vi "Main.vi"() -> ()   [LabVIEW 2018]
doc: "This template is for the Queued Message Handler design pattern.\n\nThe Event Handling Loop generates messages based on user interface actions.\n\nThe Message Handling Loop processes messages generated by the Event Handling Loop, or by other messages. The messages are string values, so new messages can be added easily to the Message Cases case structure in the Message Handling Loop. Each message cluster can also provide an optional value for Message Data, which is a variant that can be converted to whatever message-specific data is required."
uses:
  support/mqtt/Controls/QoS.ctl
  support/mqtt/Controls/Retain_Flag.ctl
  support/mqtt/Controls/DUP_Flag.ctl
  support/mqtt/Controls/Connection_Return_Codes.ctl
  controls/UI Data.ctl
  controls/App Data.ctl
  support/viewer/controls/viewewr_bus.ctl
  controls/Subscriber Data.ctl
  controls/Subscriber Comms Refs.ctl
  support/Message Queue/Message Cluster.ctl
  controls/Subscription.ctl
  support/mqtt/Controls/Connect_Flags.ctl
  support/Message Queue/Enqueue Message (Single).vi
  <vilib>/Utility/error.llb/Error Cluster From Error Code.vi
  <vilib>/ErrorRing/Error Ring.xnode
  support/Message Queue/Message Queue.lvlib
  support/User Event - Stop/User Event - Stop.lvlib
  support/mqtt/MQTT_Functions.lvlib
  support/viewer/TopicViewer.lvlib
panel:
  out "String":string
  in  "Combo Box 2":string(combo)="test/CPU/CPUcommand"
  in  "configuration file path":path=path "D:/James Pratice LV/MQTT.ini"
  in  "Key Name":string="Topics"
  in  "Section Name":string="Publish Topic"
  in  "Subscribe  list":string(combo)="test/CPU/CPUcommand"
  in  "Connect Meta":T4={"QoS"=enum."At most once", "DUP"=FALSE, "Retain"=FALSE, "Keep Alive (sec)"=60}
  in  "Tab Control":T5(tab)=enum."Subscribe"
  in  "Command":string="LabVIEW says it's "
  in  "Publish Meta":cluster{"QoS":T1, "Retain":T3, "DUP":T2}
  in  "mqtt_publish":bool
  in  "mqtt|_sendTopic":string="home/garden/fountain"
  out "Message ID (acknowledged)":u16=10
  out "all messge types":string
  in  "Clear Console":bool
  in  "mqtt_unsubscribe":bool
  in  "QoS":T1
  in  "mqtt_subscribeTopic":string(combo)="test/CPU/CPUcommand"
  in  "mqtt_subscribe":bool
  out "Console  - All Topics":string
  out "Active subscriptions":string
  out "unSubID":u16=4
  out "unsubOk":bool=TRUE
  out "subID":u16=2
  out "Granted QoS Levels":T1[](array[typedef])=[enum."At most once", enum."Exactly once", enum."At most once"]
  out "reserved count":i32
  out "Error":bool
  out "Connection Status":T6
  out "Acknowledged":bool
  out "Subscribed":bool
  out "Connected":bool=TRUE
  out "Keep Alive timer sec":dbl=4.544839382171631 caption="Elapsed Time (s)"
  in  "Exit":bool
  out "Last pingresp":bool
  in  "Message Period (ms)":i32=-1 caption="Message Period (ms) - change to -1 to turn off automated messages"
  in  "AM Command":string="LabVIEW says the time is - " caption="Command (will be a prefix to the current system time)"
  in  "AM Topic":string="home/garden/timer" caption="Topic"
  in  "AM Publish Meta":cluster{"QoS":T1, "Retain":T3, "DUP":T2} caption="Publish Meta"
  in  "mqtt_disconnect":bool
  in  "mqtt_connect":bool
  in  "Client ID":string="LVSubscribeClient1"
  in  "port":u16=1883
  in  "address (IP)":string="192.168.86.199"
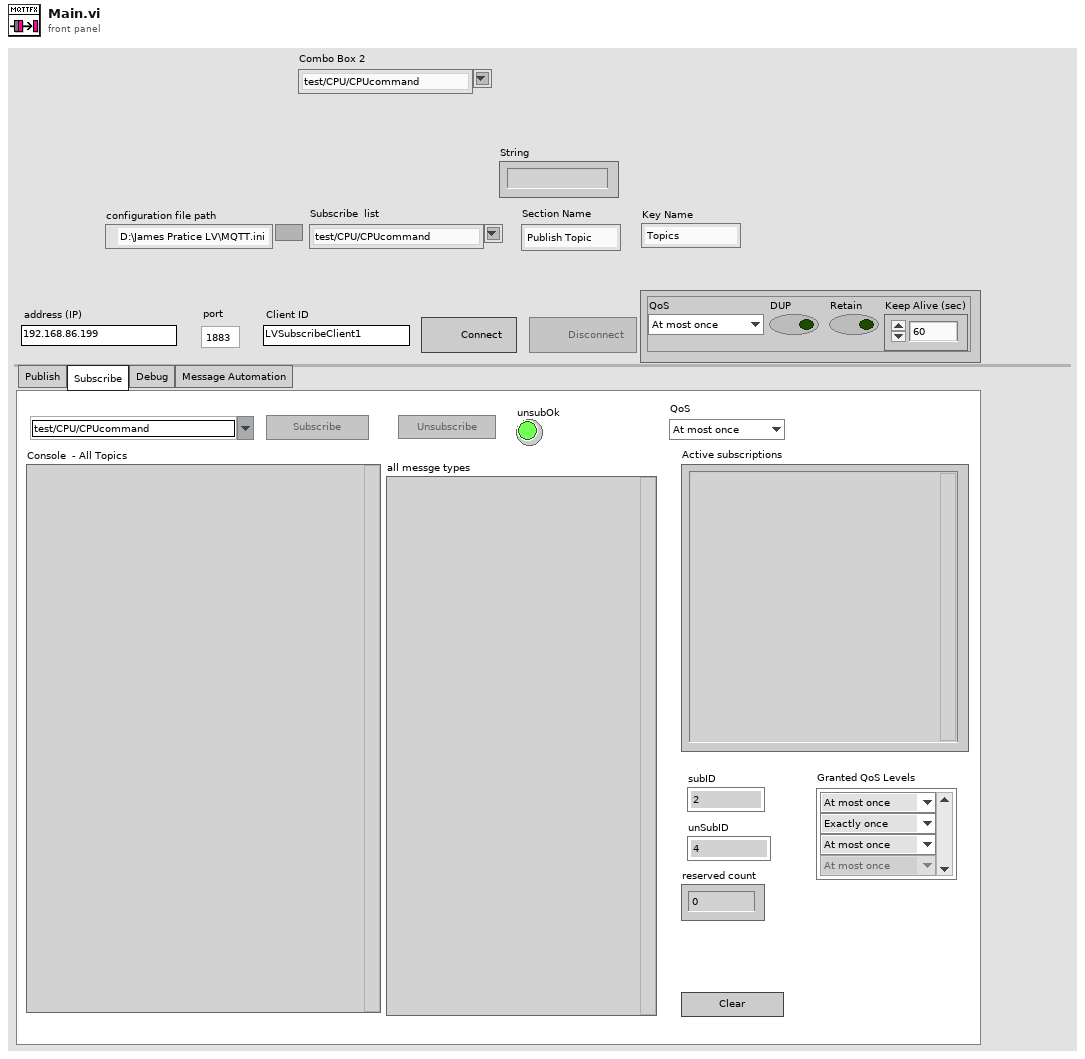
[diagram p1: front panel]
types:
  T1 = typedef "MQTT_Functions.lvlib/QoS.ctl" = enum8{"At most once", "At least once", "Exactly once", "Reserved"}
  T2 = typedef "MQTT_Functions.lvlib/DUP_Flag.ctl" = bool
  T3 = typedef "MQTT_Functions.lvlib/Retain_Flag.ctl" = bool
  T4 = cluster{"QoS":T1, "DUP":T2, "Retain":T3, "Keep Alive (sec)":u16}
  T5 = enum32{"Publish", "Subscribe", "Debug", "Message Automation"}
  T6 = typedef "MQTT_Functions.lvlib/Connection_Return_Codes.ctl" = enum16{"Connection accepted", "Connection refused: unacceptable protocol version", "Connection refused: identifier rejected", "Connection refused: Server unavailable", "Connection refused: bad user name or password", "Connection refused: not authorized"}
  T7 = typedef "Subscriber Comms Refs.ctl" = cluster{"SubscribeQ":refnum<queue>, "Subscriber Notifier":refnum<notifier>}
  T8 = typedef "Subscriber Data.ctl" = cluster{"tcpConnID":refnum<k5>, "subscriptionList":string[], "Subscribed":bool, "Keep Alive (sec)":u16, "Connected":bool, "ViewerRef":T9[], "PacketId":u16}
  T9 = typedef "TopicViewer.lvlib/viewewr_bus.ctl" = cluster{"Topic":refnum<queue>, "Stop":refnum<notifier>, "TopicName":string, "vi reference":refnum<vi>, "StopAck":refnum<notifier>}
  T10 = typedef "App Data.ctl" = cluster{"tcpConnID":refnum<k5>, "subscriptionList":string[], "Connected":bool, "Keep Alive (sec)":u16, "ViewerRef":T9[], "PacketId":u16}
  T11 = typedef "UI Data.ctl" = cluster{"Connect":refnum<vi>, "Disconnect":refnum<vi>, "Subscribe":refnum<vi>, "Unsubscribe":refnum<vi>, "Publish":refnum<vi>}
  T12 = typedef "Message Queue.lvlib/All Message Queues.ctl" = cluster{"UI":refnum<queue>, "SubscribeQ":refnum<queue>}
  T13 = cluster{"connection ID out":refnum<k5>, "Keep Alive (sec)":u16}
  T14 = typedef "TopicViewer.lvlib/Subscription.ctl" = cluster{"subscriptionInfo":cluster{"mqtt_subscribeTopic":string, "QoS":T1}, "ViewerRef":T9}
  T15 = typedef "MQTT_Functions.lvlib/MessageType.ctl" = enum32{"Reserved", "CONNECT", "CONNACK", "PUBLISH", "PUBACK", "PUBREC", "PUBREL", "PUBCOMP", "SUBSCRIBE", "SUBACK", "UNSUBSCRIBE", "UNSUBACK", "PINGREQ", "PINGRESP", "DISCONNECT", "Reserved2"}
  T16 = cluster{"mqtt_subscribeTopic":string, "QoS":T1}[]
  T17 = enum8{"Enabled", "Disabled", "Disabled and Grayed Out"}
  T18 = enum8{"Enabled", "Disabled", "Disabled and Grayed Out"}[]
  T19 = typedef "MQTT_Functions.lvlib/Connect_Flags.ctl" = cluster{"user name":bool, "password":bool, "will retain":bool, "will flag":bool, "clean session":bool, "reserved":bool, "will QoS":T1}
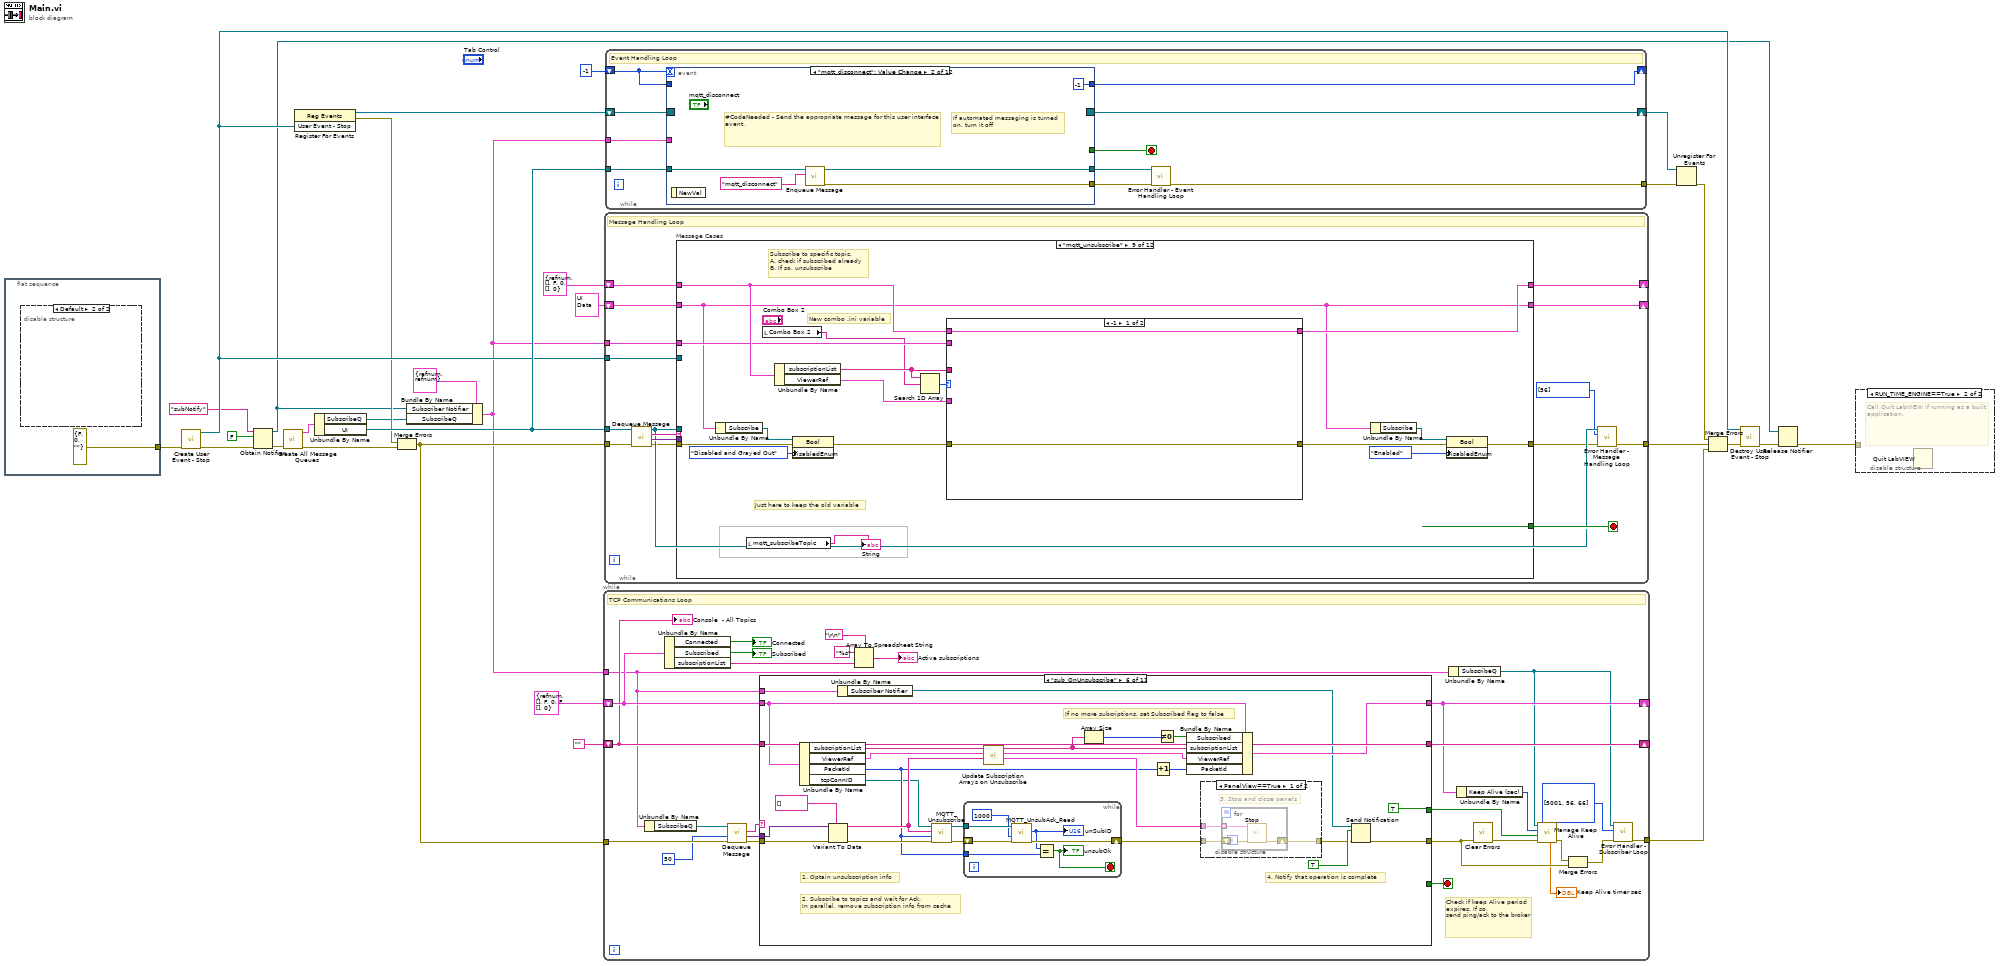
[diagram p0: block diagram]
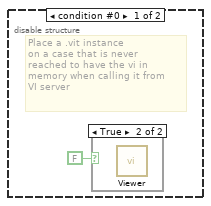
[diagram p2: hidden frame]
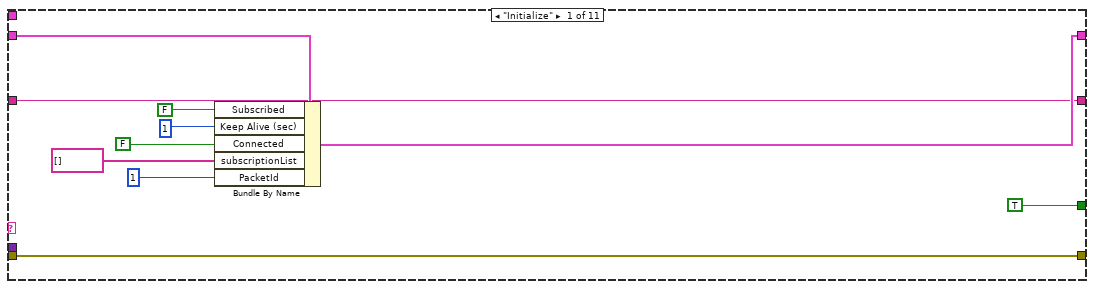
[diagram p4: hidden frame]
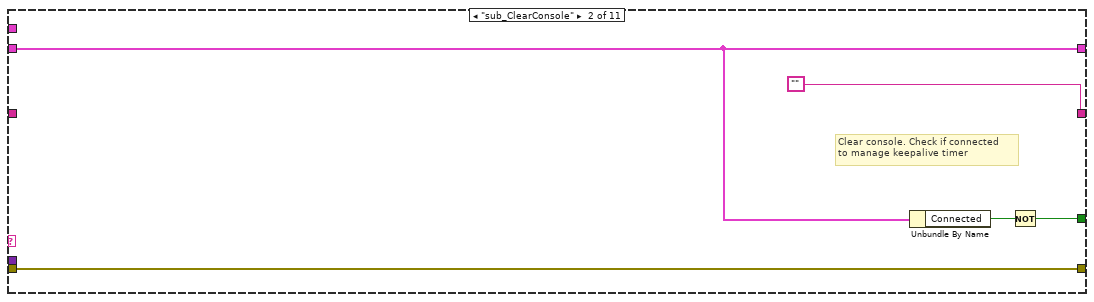
[diagram p5: hidden frame]
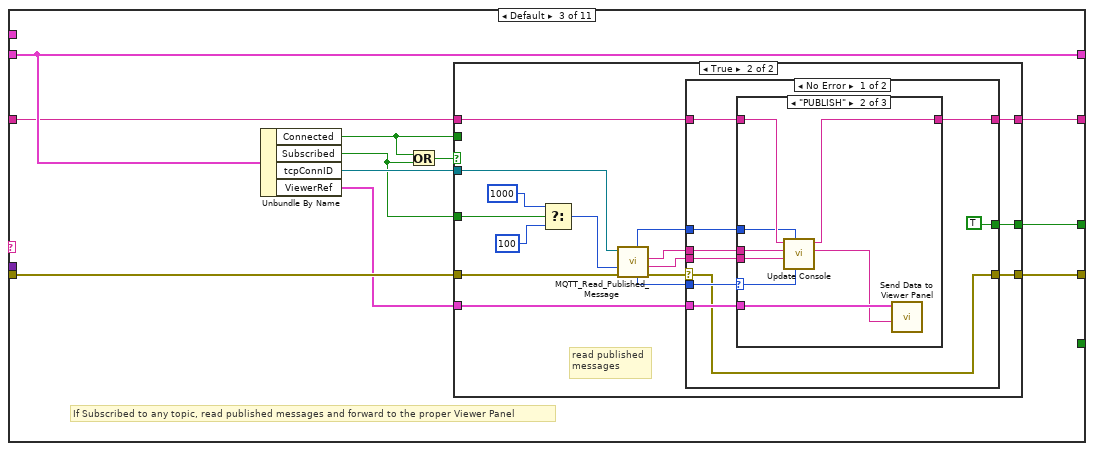
[diagram p6: hidden frame]
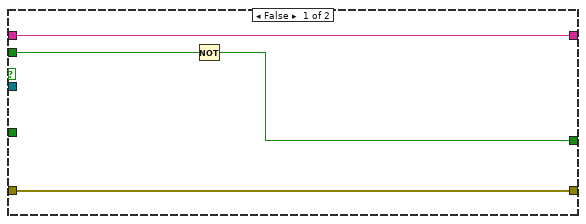
[diagram p7: hidden frame]
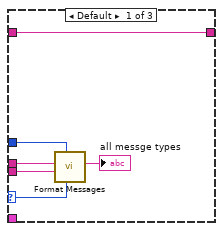
[diagram p8: hidden frame]
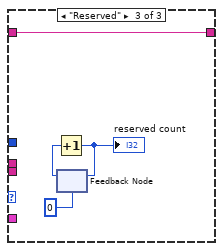
[diagram p9: hidden frame]
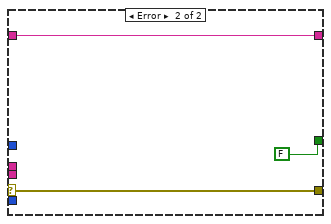
[diagram p10: hidden frame]
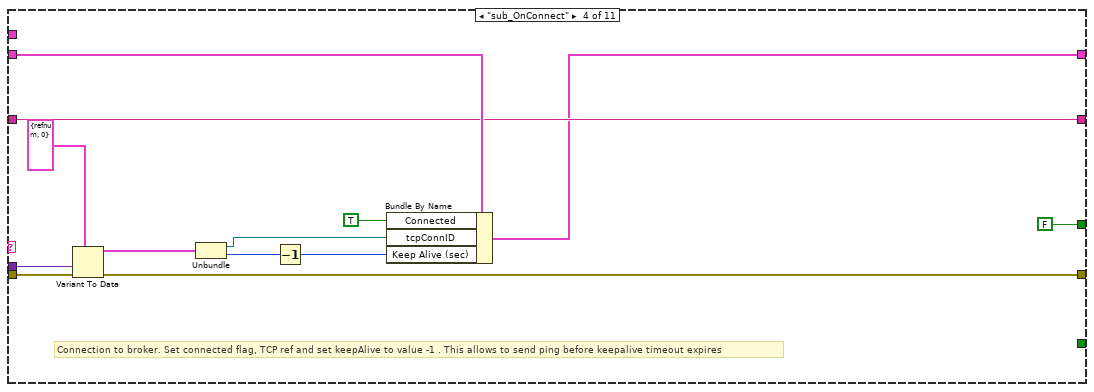
[diagram p11: hidden frame]
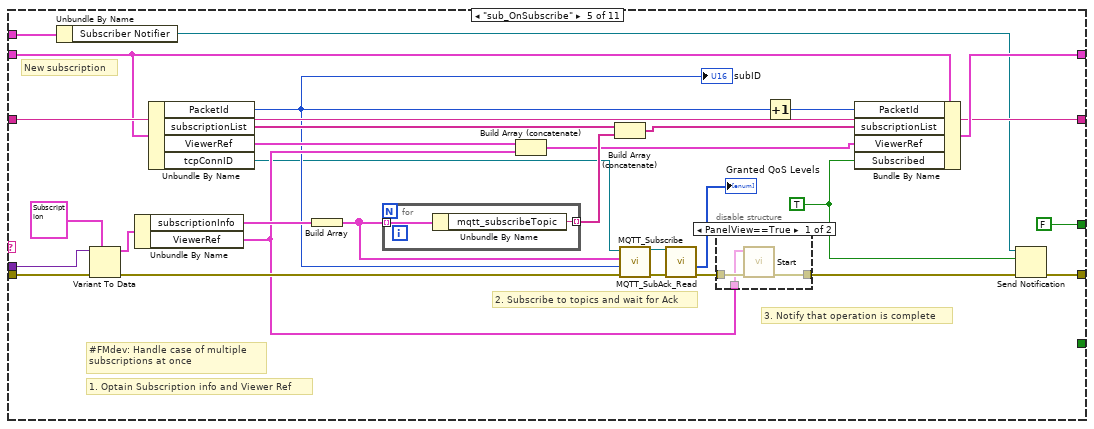
[diagram p12: hidden frame]
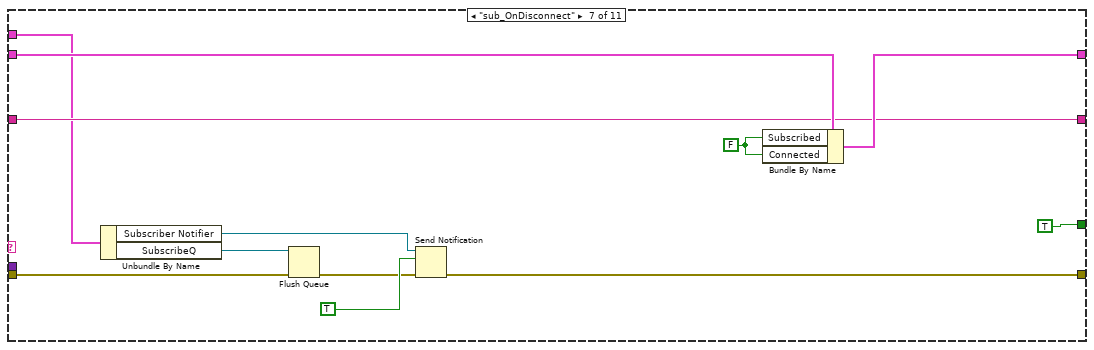
[diagram p15: hidden frame]
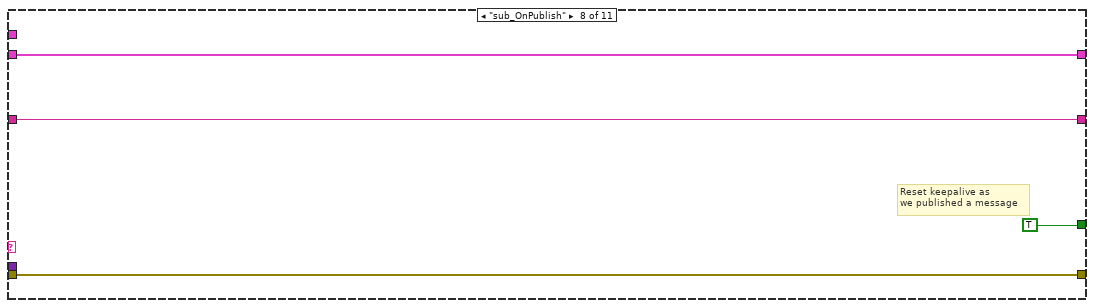
[diagram p16: hidden frame]
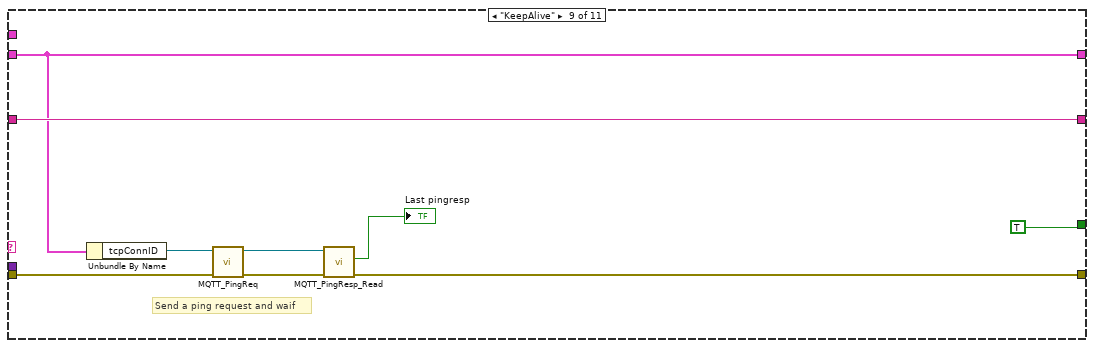
[diagram p17: hidden frame]
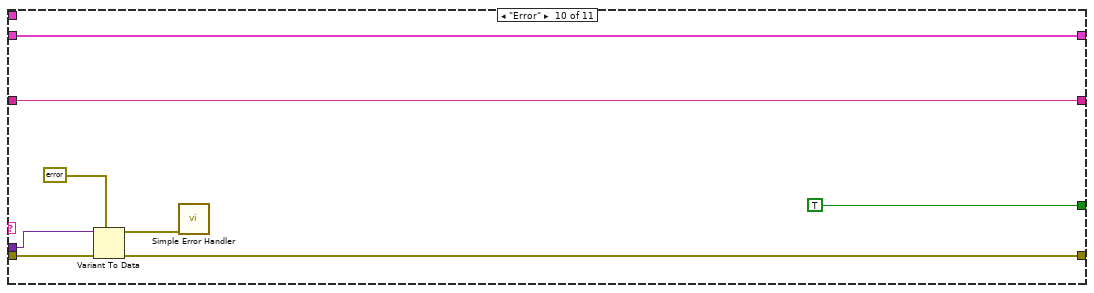
[diagram p18: hidden frame]
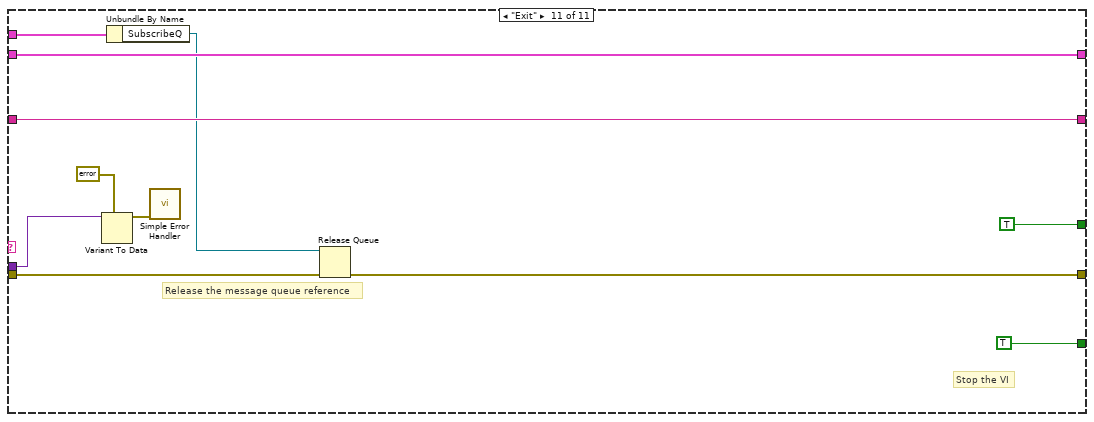
[diagram p19: hidden frame]
diagram:
  n1 = flat-sequence {
    tunnel: [errorcluster {"status"=FALSE, "code"=0, "source"=""} ("error in (no error)")] -> w6
    frame #0 {
      n2 = disable-structure shown="Default" {
        frame condition #0 {
          # "Place a .vit instance \non a case that is never\nreached to have the vi in\nmemory when calling it from \nVI server"
          n3 = case shown="True" FALSE {
            frame False {
            }
            frame True {
              n4 = call "Viewer.vi"() -> ()  [unwired: 11 in, 1 out]
            }
          }
        }
        frame condition #1 (active) {
        }
      }
    }
  }
  n5 = call "Create User Event - Stop.vi"("error in (no error)"=w6) -> ("error out"=w12:errorcluster, "User Event - Stop"=w19:refnum<user-event>)  [unwired: 9 in]
  n6 = Obtain Notifier(name (unnamed)="subNotify", notification data type=FALSE, error in (no error)=w12) -> (notifier out=w5:refnum<notifier>, error out=w11:errorcluster)  [unwired: 1 in, 1 out]
  n7 = call "Create All Message Queues.vi"("error in (no error)"=w11) -> ("error out"=w29:errorcluster, "Message Queues out"=w28:T12)  [unwired: 9 in]
  n8 = register-events(w19) -> (reference out=w20:refnum<event-registration>, error out=w18:errorcluster)  [unwired: 2 in]
  n9 = Unbundle By Name(w28) -> ("SubscribeQ"=w2:refnum<queue>, "UI"=w26:refnum<queue>)
  n10 = Merge Errors(w18, w29) -> (w16:errorcluster)
  n11 = Bundle By Name(cluster=T7 {"SubscribeQ"=refnum, "Subscriber Notifier"=refnum}, "Subscriber Notifier"=w5, "SubscribeQ"=w2) -> (w3:T7)
  n12 = while {
    tunnel: w16 -> [w59]
    shift-right: [w39] -> _
    shift-left: T8 {"tcpConnID"=refnum, "subscriptionList"=[], "Subscribed"=FALSE, "Keep Alive (sec)"=0, "Connected"=FALSE, "ViewerRef"=[], "PacketId"=0} ("App Data") -> [w37]
    tunnel: [w54] -> w14
    shift-right: [w46] -> _
    shift-left: "" -> [w36]
    tunnel: w3 -> [w32]
    stop <- w55 stop-if-true
    # "Check if keep Alive period expires. If so, \nsend ping/ack to the broker"
    # "TCP Communications Loop"
    n13 = Unbundle By Name(w32) -> ("SubscribeQ"=w34:refnum<queue>)
    n14 = Unbundle By Name(w37) -> ("Connected"=→"Connected":bool, "Subscribed"=→"Subscribed":bool, "subscriptionList"=w45:string[])
    n15 = call "Dequeue Message.vi"("error in (no error)"=w59, "timeout in ms (-1)"=50, "Message Queue"=w34) -> ("error out"=w57:errorcluster, "Message Data"=w56:variant, "Message"=w58:string)  [unwired: 5 in, 1 out]
    n16 = case shown="\"sub_OnUnsubscribe\"" w58 {
      tunnel: w57 -> [w68 w74 w83 w146 w171 w209 w233 w237 w248 w254 w264]
      tunnel: w56 -> [_ _ _ w145 w170 w206 _ _ _ w252 w266]
      tunnel: [_ _ _ _ _ _ _ _ _ _ TRUE] -> w55
      tunnel: w37 -> [w69 w72 w85 w148 w168 w200 w236 w240 w247 w257 w263]
      tunnel: [w67 w72 w85 w144 w177 w197 w235 w240 w247 w257 w263] -> w39
      tunnel: [w68 w74 w79 w142 w174 w207 w230 w237 w242 w253 w262] -> w41
      tunnel: w36 -> [w65 _ w82 w147 w176 w210 w234 w239 w249 w251 w261]
      tunnel: [w65 "" w81 w147 w176 w210 w234 w239 w249 w251 w261] -> w46
      tunnel: [TRUE w70 w78 FALSE FALSE TRUE TRUE TRUE TRUE TRUE TRUE] -> w51
      tunnel: w32 -> [_ _ _ _ w150 w185 w227 _ _ _ w259]
      frame "Initialize" {
        n17 = Bundle By Name(cluster=w69, "Subscribed"=FALSE ("Connected"), "Keep Alive (sec)"=u16 1, "Connected"=FALSE, "subscriptionList"=string[] [], "PacketId"=u16 1) -> (w67:T8)
      }
      frame "sub_ClearConsole" {
        # "Clear console. Check if connected\nto manage keepalive timer"
        n18 = Unbundle By Name(w72) -> ("Connected"=w71:bool)
        n19 = Not(x=w71) -> (.not. x?=w70:bool)
      }
      frame Default {
        # "If Subscribed to any topic, read published messages and forward to the proper Viewer Panel"
        n20 = Unbundle By Name(w85) -> ("Connected"=w77:bool, "Subscribed"=w76:bool, "tcpConnID"=w84:refnum<k5>, "ViewerRef"=w80:T9[])
        n21 = Or(x=w77, y=w76) -> (x .or. y?=w75:bool)
        n22 = case shown="True" w75 {
          tunnel: w84 -> [_ w102]
          tunnel: w83 -> [w88 w101]
          tunnel: w82 -> [w89 w100]
          tunnel: [w89 w99] -> w81
          tunnel: [w88 w94] -> w79
          tunnel: w80 -> [_ w98]
          tunnel: [w87 w95] -> w78
          tunnel: w77 -> [w86 _]
          tunnel: w76 -> [_ w93]
          frame False {
            n23 = Not(x=w86) -> (.not. x?=w87:bool)
          }
          frame True {
            # "read published\nmessages"
            n24 = Select(t=1000 ("timeout ms (25000)"), s=w93, f=100 ("timeout ms (25000)")) -> (s? t:f=w90:i32)
            n25 = call "MQTT_Read_Published_Message.vi"("error in (no error)"=w101, "timeout ms (25000)"=w90, "connection ID"=w102) -> ("error out"=w96:errorcluster, "Message"=w104:string, "Topic Name"=w105:string, "MessageType"=w103:T15, "Message ID"=w97:u16)  [unwired: 3 in, 1 out]
            n26 = case shown="No Error" w96 {
              selector: w96 -> [w106 w133]
              tunnel: w105 -> [w114 _]
              tunnel: w104 -> [w113 _]
              tunnel: w103 -> [w112 _]
              tunnel: w100 -> [w111 w134]
              tunnel: [w110 w134] -> w99
              tunnel: w98 -> [w109 _]
              tunnel: w97 -> [w108 _]
              tunnel: [TRUE FALSE] -> w95
              tunnel: [w106 w133] -> w94
              frame No Error {
                n27 = case shown="\"PUBLISH\"" w112 {
                  selector: w112 -> [w116 w121 _]
                  tunnel: w111 -> [w120 w127 w129]
                  tunnel: w114 -> [w119 w124 _]
                  tunnel: w113 -> [w118 w123 _]
                  tunnel: [w120 w126 w129] -> w110
                  tunnel: w109 -> [_ w128 _]
                  tunnel: w108 -> [w115 w122 _]
                  frame Default {
                    n28 = call "Format Messages.vi"("MessageType"=w116, "Message ID"=w115, "Message"=w118, "Topic Name"=w119) -> ("Message String"=→"all messge types":string)  [unwired: 7 in]
                  }
                  frame "PUBLISH" {
                    n29 = call "Update Console.vi"("MessageType"=w121, "Message ID"=w122, "Message"=w123, "Topic Name"=w124, "Console In"=w127) -> ("Message String"=w125:string, "Console Out"=w126:string)  [unwired: 5 in]
                    n30 = call "Send Data to Viewer Panel.vi"("Message String"=w125, "ViewerRef Array"=w128) -> ()  [unwired: 10 in]
                  }
                  frame "Reserved" {
                    n31 = feedback #1(0) -> (w131:i32)
                    n32 = Increment(x=w131) -> (x+1=w130:i32)
                    "reserved count" <- w130
                    n33 = feedback-in #1(w130) -> ()
                  }
                }
              }
              frame Error {
              }
            }
          }
        }
      }
      frame "sub_OnConnect" {
        # "Connection to broker. Set connected flag, TCP ref and set keepAlive to value -1 . This allows to send ping before keepalive timeout expires"
        n34 = Variant To Data(error in=w146, type=T13 {"connection ID out"=refnum, "Keep Alive (sec)"=0} ("output cluster"), Variant=w145) -> (data=w139:T13, error out=w142:errorcluster)
        n35 = Unbundle(w139) -> ("connection ID out"=w138:refnum<k5>, "Keep Alive (sec)"=w137:u16)
        n36 = Decrement(x=w137) -> (x-1=w136:u16)
        n37 = Bundle By Name(cluster=w148, "Connected"=TRUE, "tcpConnID"=w138, "Keep Alive (sec)"=w136) -> (w144:T8)
      }
      frame "sub_OnSubscribe" {
        w154 = TRUE ("notification")
        # "3. Notify that operation is complete"
        # "2. Subscribe to topics and wait for Ack"
        # "#FMdev: Handle case of multiple\nsubscriptions at once"
        # "1. Optain Subscription info and Viewer Ref"
        # "New subscription"
        n38 = Unbundle By Name(w150) -> ("Subscriber Notifier"=w149:refnum<notifier>)
        n39 = Variant To Data(error in=w171, type=T14 {"subscriptionInfo"={"mqtt_subscribeTopic"="", "QoS"=enum."At most once"}, "ViewerRef"={"Topic"=refnum, "Stop"=refnum, "TopicName"="", "vi reference"=refnum, "StopAck"=refnum}}, Variant=w170) -> (data=w163:T14, error out=w169:errorcluster)
        n40 = Unbundle By Name(w163) -> ("subscriptionInfo"=w162:cluster{"mqtt_subscribeTopic":string, "QoS":T1}, "ViewerRef"=w157:T9)
        n41 = Unbundle By Name(w168) -> ("PacketId"=w153:u16, "subscriptionList"=w167:string[], "ViewerRef"=w160:T9[], "tcpConnID"=w151:refnum<k5>)
        "subID" <- w153
        n42 = Build Array(w162) -> (w161:T16)
        n43 = for {
          tunnel: w161 -> [w183] mode=indexing
          tunnel: [w182] -> w166 mode=indexing
          n44 = Unbundle By Name(w183) -> ("mqtt_subscribeTopic"=w182:string)
        }
        n45 = Build Array (concatenate)(w160, w157) -> (w159:T9[])
        n46 = Build Array (concatenate)(w167, w166) -> (w165:string[])
        n47 = call "MQTT_Subscribe.vi"("error in (no error)"=w169, "Message ID"=w153, "Subscription Info Array"=w161, "connection ID"=w151) -> ("error out"=w173:errorcluster, "connection ID out"=w172:refnum<k5>)  [unwired: 6 in]
        n48 = call "MQTT_SubAck_Read.vi"("error in (no error)"=w173, "connection ID"=w172) -> ("error out"=w158:errorcluster, "Granted QoS Levels"=→"Granted QoS Levels":T1[])  [unwired: 7 in, 1 out]
        n49 = disable-structure shown="PanelView==True" {
          disable-tunnel: w158 -> [w180 w181]
          disable-tunnel: w157 -> [w179 _]
          disable-tunnel: [w178 w181] -> w156
          frame condition #0 {
            n50 = call "Start.vi"("error in (no error)"=w180, "ViewerRef"=w179) -> ("error out"=w178:errorcluster)  [unwired: 9 in]
          }
          frame condition #1 (active) {
          }
        }
        n51 = Increment(x=w153) -> (x+1=w152:u16)
        n52 = Bundle By Name(cluster=w168, "PacketId"=w152, "subscriptionList"=w165, "ViewerRef"=w159, "Subscribed"=w154) -> (w177:T8)
        n53 = Send Notification(notification=w154, notifier=w149, error in (no error)=w156) -> (error out=w174:errorcluster)  [unwired: 1 out]
      }
      frame "sub_OnUnsubscribe" {
        # "If no more subcriptions, set Subscribed flag to false"
        # "2. Subscribe to topics and wait for Ack.\nIn parallel, remove subscription info from cache"
        # "1. Optain unsubscription info"
        # "4. Notify that operation is complete"
        n54 = Unbundle By Name(w200) -> ("subscriptionList"=w202:string[], "ViewerRef"=w188:T9[], "PacketId"=w189:u16, "tcpConnID"=w186:refnum<k5>)
        n55 = Variant To Data(error in=w209, type=string[] [] ("UnSubscribe Topic Array"), Variant=w206) -> (data=w201:string[], error out=w190:errorcluster)
        n56 = Unbundle By Name(w185) -> ("Subscriber Notifier"=w184:refnum<notifier>)
        n57 = call "MQTT_Unsubscribe.vi"("error in (no error)"=w190, "Message ID"=w189, "UnSubscribe Topic Array"=w201, "connection ID"=w186) -> ("error out"=w205:errorcluster, "connection ID out"=w204:refnum<k5>)  [unwired: 5 in, 1 out]
        n58 = while {
          tunnel: w204 -> [w216]
          tunnel: w189 -> [w212]
          shift-right: [w214] -> w194
          shift-left: w205 -> [w217]
          stop <- w211 stop-if-true
          n59 = call "MQTT_UnsubAck_Read.vi"("error in (no error)"=w217, "timeout ms (25000)"=1000, "connection ID"=w216) -> ("error out"=w214:errorcluster, "MessageID"=w213:u16)  [unwired: 6 in, 1 out]
          "unSubID" <- w213
          n60 = Equal?(x=w213, y=w212) -> (x = y?=w211:bool)
          "unsubOk" <- w211
        }
        n61 = call "Update Subscription Arrays on Unsubscribe.vi"("UnSubscribe Topic Array"=w201, "ViewerRef in"=w188, "subscriptionList in"=w202) -> ("ViewerRef's to close"=w192:T9[], "ViewerRef out"=w195:T9[], "subscriptionList out"=w199:string[])  [unwired: 6 in]
        n62 = Array Size(array=w199) -> (size(s)=w198:i32)
        n63 = Increment(x=w189) -> (x+1=w191:u16)
        n64 = Not Equal To 0?(x=w198) -> (x != 0?=w187:bool)
        n65 = Bundle By Name(cluster=w200, "Subscribed"=w187, "subscriptionList"=w199, "ViewerRef"=w195, "PacketId"=w191) -> (w197:T8)
        n66 = disable-structure shown="PanelView==True" {
          disable-tunnel: w194 -> [w220 w224]
          disable-tunnel: [w219 w224] -> w193
          disable-tunnel: w192 -> [w218 _]
          frame condition #0 {
            # "3. Stop and close panels"
            n67 = for {
              tunnel: w218 -> [w221] mode=indexing
              shift-right: [w222] -> w219
              shift-left: w220 -> [w223]
              n68 = call "Stop.vi"("error in (no error)"=w223, "ViewerRef"=w221) -> ("error out"=w222:errorcluster)  [unwired: 9 in]
            }
          }
          frame condition #1 (active) {
          }
        }
        n69 = Send Notification(notification=TRUE, notifier=w184, error in (no error)=w193) -> (error out=w207:errorcluster)  [unwired: 1 out]
      }
      frame "sub_OnDisconnect" {
        w228 = FALSE ("Subscribed")
        n70 = Unbundle By Name(w227) -> ("Subscriber Notifier"=w226:refnum<notifier>, "SubscribeQ"=w225:refnum<queue>)
        n71 = Flush Queue(queue=w225, error in (no error)=w233) -> (error out=w231:errorcluster)  [unwired: 2 out]
        n72 = Send Notification(notification=TRUE, notifier=w226, error in (no error)=w231) -> (error out=w230:errorcluster)  [unwired: 1 out]
        n73 = Bundle By Name(cluster=w236, "Subscribed"=w228, "Connected"=w228) -> (w235:T8)
      }
      frame "sub_OnPublish" {
        # "Reset keepalive as \nwe published a message"
      }
      frame "KeepAlive" {
        # "Send a ping request and waif"
        n74 = Unbundle By Name(w247) -> ("tcpConnID"=w246:refnum<k5>)
        n75 = call "MQTT_PingReq.vi"("error in (no error)"=w248, "connection ID"=w246) -> ("error out"=w243:errorcluster, "connection ID out"=w244:refnum<k5>)  [unwired: 7 in, 1 out]
        n76 = call "MQTT_PingResp_Read.vi"("error in (no error)"=w243, "connection ID"=w244) -> ("error out"=w242:errorcluster, "ok"=→"Last pingresp":bool)  [unwired: 7 in, 1 out]
      }
      frame "Error" {
        n77 = Variant To Data(error in=w254, type=errorcluster {"status"=FALSE, "code"=0, "source"=""} ("error constant"), Variant=w252) -> (data=w256:errorcluster, error out=w253:errorcluster)
        n78 = call <vilib>:"Simple Error Handler.vi"("error in (no error)"=w256) -> ()  [unwired: 4 in, 5 out]
      }
      frame "Exit" {
        # "Release the message queue reference"
        # "Stop the VI"
        n79 = Variant To Data(type=errorcluster {"status"=FALSE, "code"=0, "source"=""} ("error constant"), Variant=w266) -> (data=w267:errorcluster)  [unwired: 1 in, 1 out]
        n80 = Unbundle By Name(w259) -> ("SubscribeQ"=w258:refnum<queue>)
        n81 = call <vilib>:"Simple Error Handler.vi"("error in (no error)"=w267) -> ()  [unwired: 4 in, 5 out]
        n82 = Release Queue(queue=w258, error in (no error)=w264) -> (error out=w262:errorcluster)  [unwired: 1 in, 2 out]
      }
    }
    n83 = Array To Spreadsheet String(delimiter (Tab)="\r\n", array=w45, 3:"%s" ("format string")) -> (spreadsheet string=→"Active subscriptions":string)
    n84 = Unbundle By Name(w32) -> ("SubscribeQ"=w33:refnum<queue>)
    n85 = Unbundle By Name(w39) -> ("Keep Alive (sec)"=w38:u16)
    n86 = call <vilib>:"Clear Errors.vi"("error in (no error)"=w41) -> ("error out"=w44:errorcluster)  [unwired: 5 in, 1 out]
    n87 = call "Manage Keep Alive.vi"("error in (no error)"=w44, "Reset Keepalive"=w51, "Keep Alive (sec)"=w38, "SubscriberQ"=w33) -> ("error out"=w43:errorcluster, "Elapsed Time (s)"=→"Keep Alive timer sec":dbl)  [unwired: 6 in]
    n88 = Merge Errors(w43, w41) -> (w42:errorcluster)
    n89 = call "Error Handler - Subscriber Loop.vi"("error in (no error)"=w42, "Ignore Errors (Runtime)"=i32[] [5001, 56, 66], "Message Queue"=w33) -> ("dup error in"=w54:errorcluster)  [unwired: 7 in, 1 out]
    "Console  - All Topics" <- w36
  }
  n90 = while {
    tunnel: w26 -> [w277]
    shift-right: [w283] -> _
    shift-left: T11 {"Connect"=refnum, "Disconnect"=refnum, "Subscribe"=refnum, "Unsubscribe"=refnum, "Publish"=refnum} ("Data Cluster") -> [w284]
    tunnel: w19 -> [w281]
    tunnel: w16 -> [w280]
    tunnel: [w275] -> w27
    shift-right: [w272] -> _
    shift-left: T10 {"tcpConnID"=refnum, "subscriptionList"=[], "Connected"=FALSE, "Keep Alive (sec)"=0, "ViewerRef"=[], "PacketId"=0} -> [w273]
    tunnel: w3 -> [w269]
    stop <- w282 stop-if-true
    # "Message Handling Loop"
    n91 = call "Dequeue Message.vi"("error in (no error)"=w280, "Message Queue"=w277) -> ("error out"=w270:errorcluster, "Message Data"=w278:variant, "Message"=w279:string, "dup Message Queue"=w276:refnum<queue>)  [unwired: 6 in]
    n92 = case "Message Cases" shown="\"mqtt_unsubscribe\"" w279 {
      selector: w279 -> [_ _ _ _ _ _ _ _ _ _ _ w571]
      tunnel: w276 -> [_ _ _ w324 _ _ _ _ _ _ w569 _]
      tunnel: w270 -> [w288 w306 w316 w323 w349 w397 w423 w454 w502 w540 w562 _]
      tunnel: [w287 w304 w310 w322 w334 w386 w414 w457 w494 w536 w565 w572] -> w274
      tunnel: w284 -> [w301 w308 w315 w325 w340 w389 w425 w453 w493 w541 w568 w573]
      tunnel: [w289 w308 w315 w325 w339 w389 w425 w452 w493 w541 w568 w573] -> w283
      tunnel: [_ _ _ _ _ _ _ _ _ _ TRUE _] -> w282
      tunnel: w278 -> [_ _ w314 _ _ _ _ _ _ _ w559 _]
      tunnel: w281 -> [_ _ _ _ _ _ _ _ _ _ w564 _]
      tunnel: w273 -> [w300 w307 w309 w321 w341 w384 w424 w459 w507 w539 w558 w570]
      tunnel: [w299 w307 w309 w321 w342 w396 w411 w458 w506 w538 w558 w570] -> w272
      tunnel: w269 -> [_ w303 _ _ w333 w385 w406 w451 w501 w533 _ _]
      frame "Initialize" {
        w285 = T18 [enum."Enabled", enum."Disabled and Grayed Out", enum."Disabled and Grayed Out", enum."Disabled and Grayed Out", enum."Disabled and Grayed Out"] items=["Enabled", "Disabled", "Disabled and Grayed Out"] ("State Array")
        w286 = ""
        w291 = FALSE ("Subscribed")
        # "Initialize local variables"
        # "Initialize buttons"
        # "#FMdev: 1) Vi server to manage UI"
        # "Initialize - All initialization work should take place in this message, since other loops can potentially enqueue messages that execute immediately after this one."
        n93 = control-ref of="mqtt_connect"() -> (w297:refnum<vi>)
        n94 = control-ref of="mqtt_disconnect"() -> (w296:refnum<vi>)
        n95 = control-ref of="mqtt_subscribe"() -> (w295:refnum<vi>)
        n96 = control-ref of="mqtt_unsubscribe"() -> (w294:refnum<vi>)
        n97 = control-ref of="mqtt_publish"() -> (w292:refnum<vi>)
        n98 = Bundle By Name(cluster=w301, "Connect"=w297, "Disconnect"=w296, "Subscribe"=w295, "Unsubscribe"=w294, "Publish"=w292) -> (w289:T11)
        n99 = Bundle By Name(cluster=w300, "Connected"=FALSE, "subscriptionList"=string[] [], "PacketId"=u16 1) -> (w299:T10)
        n100 = local write "Console  - All Topics"(w286) -> ()
        n101 = local write "Active subscriptions"(w286) -> ()
        n102 = local write "Last pingresp"(w291) -> ()
        n103 = local write "Connected"(w291) -> ()
        n104 = local write "Subscribed"(w291) -> ()
        n105 = local write "Error"(w291) -> ()
        n106 = call "Enable Disable Controls.vi"("error in (no error)"=w288, "State Array"=w285, "Data Cluster"=w289) -> ("error out"=w287:errorcluster)  [unwired: 8 in]
      }
      frame "ClearConsole" {
        # "Proxy to clear console from old messages"
        n107 = Unbundle By Name(w303) -> ("SubscribeQ"=w302:refnum<queue>)
        n108 = call-poly "Enqueue Message.vi"("error in (no error)"=w306, "Message"="sub_ClearConsole", "Message Queue"=w302) -> ("error out"=w304:errorcluster)  [unwired: 7 in, 1 out]
      }
      frame "Error" {
        # "#CodeRecommended - If you ever change the name of this \"Error\" message, you'll need to update the name in the Check Loop Error.vi as well."
        # "#CodeRecommended - Consider creating a system for logging errors in some way. These errors are for notification purposes only. Handling of specific errors should be performed in the message frames that generated the error."
        # "Error - Display an error dialog. This message is sent by the \"Error Handler\" VIs at the end of other loops in this application."
        n109 = Variant To Data(error in=w316, type=errorcluster {"status"=FALSE, "code"=0, "source"=""} ("error constant"), Variant=w314) -> (data=w312:errorcluster, error out=w311:errorcluster)
        n110 = call <vilib>:"Simple Error Handler.vi"("error in (no error)"=w312) -> ()  [unwired: 4 in, 5 out]
        n111 = Merge Errors(w311) -> (w310:errorcluster)
      }
      frame "Confirm Quit" {
        # "If connected to a broker, then unsubcribe to existing topics and disconnect\nIf not connected, just exit"
        # "Confirm Quit - Message that can confirm whether or not the user wants to exit the application."
        n112 = Unbundle By Name(w321) -> ("Connected"=w320:bool)
        n113 = Select(t=string[] ["mqtt_unsubscribeAll", "mqtt_disconnect", "Exit"] ("Message"), s=w320, f=string[] ["Exit"]) -> (s? t:f=w319:string[])
        n114 = for {
          tunnel: w319 -> [w326] mode=indexing
          shift-right: [w328] -> w322
          shift-left: w323 -> [w329]
          tunnel: w324 -> [w327]
          n115 = call-poly "Enqueue Message.vi"("error in (no error)"=w329, "Message"=w326, "Message Queue"=w327) -> ("error out"=w328:errorcluster)  [unwired: 7 in, 1 out]
        }
      }
      frame "mqtt_connect" {
        w348 = T19 {"user name"=FALSE, "password"=FALSE, "will retain"=FALSE, "will flag"=FALSE, "clean session"=FALSE, "reserved"=FALSE, "will QoS"=enum."At most once"}  # Connect Flags
        # "Filter on error and then on connection status"
        # "Connect to broker using user provided\nvalue. Using default collect flags"
        n116 = Bundle("address (IP)"="address (IP)", "port"="port") -> (w344:cluster{"address (IP)":string, "port":u16})  [unwired: 1 in]
        n117 = call "MQTT_Connect.vi"("timeout ms (20000)"=10000, "Connect Meta"="Connect Meta", "Client ID"="Client ID", "Connect Flags"=w348, "error in (no error)"=w349, "MQTT Broker"=w344) -> ("error out"=w336:errorcluster, "Connection Status"=w343:T6, "connection ID out"=w331:refnum<k5>)  [unwired: 3 in]
        "Connection Status" <- w343
        n118 = Unbundle By Name("Connect Meta") -> ("Keep Alive (sec)"=w330:u16)
        n119 = Unbundle By Name(w333) -> ("SubscribeQ"=w332:refnum<queue>)
        n120 = case shown="No Error" w336 {
          selector: w336 -> [w354 w382]
          tunnel: w343 -> [w360 _]
          tunnel: [w359 w381] -> w342
          tunnel: w341 -> [w358 w381]
          tunnel: w340 -> [w357 w380]
          tunnel: [w356 w380] -> w339
          tunnel: w330 -> [w355 _]
          tunnel: [w351 w382] -> w334
          tunnel: [w353 TRUE ("Timeout")] -> w335
          tunnel: w332 -> [w352 _]
          tunnel: w331 -> [w350 _]
          frame No Error {
            n121 = case shown="\"Connection accepted\", Default" w360 {
              tunnel: w358 -> [w374 w378]
              tunnel: [w373 w378] -> w359
              tunnel: w357 -> [w371 w377]
              tunnel: [w371 w377] -> w356
              tunnel: w355 -> [w362 _]
              tunnel: w354 -> [w368 w376]
              tunnel: [w364 w376] -> w351
              tunnel: [FALSE ("Timeout") TRUE ("Timeout")] -> w353
              tunnel: w352 -> [w367 _]
              tunnel: w350 -> [w363 _]
              frame "Connection accepted", Default {
                w366 = T18 [enum."Disabled and Grayed Out", enum."Enabled", enum."Enabled", enum."Disabled and Grayed Out", enum."Enabled"] items=["Enabled", "Disabled", "Disabled and Grayed Out"] ("State Array")
                # "Connection accepted, change UI accordingly and send OnConnect event to\nSubscriber Loop"
                n122 = Bundle By Name(cluster=w374, "Connected"=TRUE, "Keep Alive (sec)"=w362, "tcpConnID"=w363) -> (w373:T10)
                n123 = Bundle("connection ID out"=w363, "Keep Alive (sec)"=w362) -> (w361:T13)  [unwired: 1 in]
                n124 = call-poly "Enqueue Message.vi"("error in (no error)"=w368, "Message Data"=w361, "Message"="sub_OnConnect", "Message Queue"=w367) -> ("error out"=w365:errorcluster)  [unwired: 6 in, 1 out]
                n125 = call "Enable Disable Controls.vi"("error in (no error)"=w365, "State Array"=w366, "Data Cluster"=w371) -> ("error out"=w364:errorcluster)  [unwired: 8 in]
              }
              frame "Connection refused: unacceptable protocol version" {
                # "#FM_note: manage refused connection"
              }
            }
          }
          frame Error {
            # "Error connecting. Filter specific errors later on Error Handler VI later on"
          }
        }
        "Error" <- w335
      }
      frame "mqtt_disconnect" {
        w388 = T18 [enum."Enabled", enum."Disabled and Grayed Out", enum."Disabled and Grayed Out", enum."Disabled and Grayed Out", enum."Disabled and Grayed Out"] items=["Enabled", "Disabled", "Disabled and Grayed Out"] ("State Array")
        # "Disconnect anyway and change UI accordingly"
        # "Send OnDisconnect message to subscriber loop and \nwait for operation completed (notifier received)"
        n126 = Unbundle By Name(w384) -> ("subscriptionList"=w383:string[])
        n127 = Unbundle By Name(w384) -> ("tcpConnID"=w398:refnum<k5>)
        n128 = Array Size(array=w383) -> (size(s)=w395:i32)
        n129 = case shown="0" w395 {
          tunnel: w397 -> [w399 w404]
          tunnel: [w399 w403] -> w394
          tunnel: w383 -> [_ w400]
          tunnel: w385 -> [_ w402]
          frame 0 {
          }
          frame Default {
            n130 = call "Send Msg and Wait on Response.vi"("error in (no error)"=w404, "Message Data"=w400, "Message"="sub_OnUnsubscribe", "Subscription References"=w402) -> ("error out"=w403:errorcluster)  [unwired: 7 in]
          }
        }
        n131 = call "Send Msg and Wait on Response.vi"("error in (no error)"=w394, "Message"="sub_OnDisconnect", "Subscription References"=w385) -> ("error out"=w393:errorcluster)  [unwired: 8 in]
        n132 = Bundle By Name(cluster=w384, "Connected"=FALSE, "subscriptionList"=string[] []) -> (w396:T10)
        n133 = call "MQTT_Disconnect.vi"("error in (no error)"=w393, "connection ID"=w398) -> ("error out"=w387:errorcluster)  [unwired: 9 in]
        n134 = call "Enable Disable Controls.vi"("error in (no error)"=w387, "State Array"=w388, "Data Cluster"=w389) -> ("error out"=w386:errorcluster)  [unwired: 8 in]
      }
      frame "mqtt_publish" {
        # "Send an OnPublish message to\nreset keepAlive counter on subcriber"
        # "Publish message. Depending on Quality of Service, handle ack signals"
        n135 = Unbundle By Name(w424) -> ("tcpConnID"=w422:refnum<k5>, "PacketId"=w412:u16)
        n136 = call "MQTT_Publish.vi"("Message ID"=w412, "Publish Meta"="Publish Meta", "error in (no error)"=w423, "Message to be published"="Command", "Topic"="mqtt|_sendTopic", "connection ID"=w422) -> ("error out"=w419:errorcluster, "connection ID out"=w418:refnum<k5>)  [unwired: 4 in]
        n137 = Unbundle By Name("Publish Meta") -> ("QoS"=w420:T1)
        n138 = Unbundle By Name(w406) -> ("SubscribeQ"=w405:refnum<queue>)
        n139 = case shown="\"At most once\", Default" w420 {
          tunnel: w419 -> [w428 w433 w444]
          tunnel: w418 -> [_ w434 w445]
          tunnel: [w428 w431 w438] -> w415
          tunnel: w412 -> [w426 w432 w443]
          tunnel: [FALSE w430 w439] -> w410
          tunnel: [w426 w429 w437] -> w408
          frame "At most once", Default {
            # "QoS 0: no PubACK, fire and forget"
          }
          frame "At least once" {
            # "QoS 1: PubACK"
            n140 = call "MQTT_PubAck_Read.vi"("error in (no error)"=w433, "connection ID"=w434) -> ("error out"=w431:errorcluster, "Message ID"=w429:u16)  [unwired: 7 in, 1 out]
            n141 = Equal?(x=w429, y=w432) -> (x = y?=w430:bool)
          }
          frame "Exactly once" {
            # "QoS 2: PubREC, PubREL, PubCOMP"
            n142 = call "MQTT_PubRec_Read.vi"("error in (no error)"=w444, "connection ID"=w445) -> ("error out"=w442:errorcluster, "Message ID"=w440:u16, "connection ID out"=w441:refnum<k5>)  [unwired: 7 in]
            n143 = call "MQTT_PubRel_Send.vi"("error in (no error)"=w442, "Message ID"=w440, "connection ID"=w441) -> ("error out"=w435:errorcluster, "connection ID out"=w436:refnum<k5>)  [unwired: 6 in, 1 out]
            n144 = call "MQTT_PubComp_Read.vi"("error in (no error)"=w435, "connection ID"=w436) -> ("error out"=w438:errorcluster, "Message ID"=w437:u16)  [unwired: 7 in, 1 out]
            n145 = Equal?(x=w437, y=w443) -> (x = y?=w439:bool)
          }
        }
        "Message ID (acknowledged)" <- w408
        "Acknowledged" <- w410
        n146 = Increment(x=w408) -> (x+1=w407:u16)
        n147 = Select(t=w407, s=w410, f=w408) -> (s? t:f=w409:u16)
        n148 = Bundle By Name(cluster=w424, "PacketId"=w409) -> (w411:T10)
        n149 = call-poly "Enqueue Message.vi"("error in (no error)"=w415, "Message"="sub_OnPublish", "Message Queue"=w405) -> ("error out"=w414:errorcluster)  [unwired: 7 in, 1 out]
      }
      frame "mqtt_subscribe" {
        n150 = control-ref of="Subscribe  list"() -> (w447:refnum<vi>)
        n151 = call "Fill_Combo_API_Box (SubVI).vi"("Section Name"="Section Name", "Key Name"="Key Name", "Combo Box"="Subscribe  list", "configuration file path"="configuration file path", "ComboBox in"=w447) -> ()  [unwired: 7 in]
        n152 = Unbundle By Name(w459) -> ("subscriptionList"=w460:string[], "ViewerRef"=w455:T9[])
        n153 = Bundle("Subscribe  list"="Subscribe  list", "QoS"="QoS") -> (w456:cluster{"Subscribe  list":string, "QoS":T1})  [unwired: 1 in]
        n154 = Search 1D Array(1D array=w460, element="Subscribe  list") -> (index of element=w461:i32)  [unwired: 1 in]
        n155 = case shown="-1" w461 {
          tunnel: w454 -> [w465 w479]
          tunnel: [w465 w473] -> w457
          tunnel: w456 -> [_ w480]
          tunnel: w460 -> [_ w485]
          tunnel: "Subscribe  list" -> [_ w478]
          tunnel: w459 -> [w464 w484]
          tunnel: [w464 w483] -> w458
          tunnel: w455 -> [_ w476]
          tunnel: w453 -> [w463 w474]
          tunnel: [w463 w474] -> w452
          tunnel: w451 -> [_ w468]
          frame Default {
            # "Already subscribed, don't do anything"
          }
          frame -1 {
            # "B. Send OnSubscribe message \nand wait for done"
            # "Not subscribed to this topic yet"
            n156 = disable-structure shown="PanelView==True" {
              disable-tunnel: w479 -> [w489 w490]
              disable-tunnel: w478 -> [w488 _]
              disable-tunnel: [w487 w490] -> w469
              disable-tunnel: [w486 _] -> w475
              frame condition #0 {
                # "A. Create new Viewer Panel"
                n157 = call "Create.vi"("error in (no error)"=w489, "Topic"=w488) -> ("error out"=w487:errorcluster, "ViewerRef"=w486:T9)  [unwired: 8 in]
              }
              frame condition #1 (active) {
              }
            }
            n158 = Build Array (concatenate)(w476, w475) -> (w477:T9[])
            n159 = Bundle By Name(cluster=T14 {"subscriptionInfo"={"mqtt_subscribeTopic"="", "QoS"=enum."At most once"}, "ViewerRef"={"Topic"=refnum, "Stop"=refnum, "TopicName"="", "vi reference"=refnum, "StopAck"=refnum}}, "subscriptionInfo"=w480, "ViewerRef"=w475) -> (w466:T14)
            n160 = Build Array (concatenate)(w485, w478) -> (w482:string[])
            n161 = Bundle By Name(cluster=w484, "subscriptionList"=w482, "ViewerRef"=w477) -> (w483:T10)
            n162 = call "Send Msg and Wait on Response.vi"("error in (no error)"=w469, "Message Data"=w466, "Message"="sub_OnSubscribe", "Subscription References"=w468) -> ("error out"=w470:errorcluster)  [unwired: 7 in]
            n163 = Unbundle By Name(w474) -> ("Unsubscribe"=w472:refnum<vi>)
            n164 = property class="Bool"(reference=w472, error in=w470, "DisabledEnum"=T17."Enabled" ("Disabled")) -> (error out=w473:errorcluster)  [unwired: 1 out]
          }
        }
      }
      frame "mqtt_unsubscribe" {
        # "New combo .ini variable"
        # "Just here to keep the old variable"
        # "Subscribe to specific topic.\nA. check if subscribed already\nB. If so, unsubscribe"
        n165 = Unbundle By Name(w493) -> ("Subscribe"=w499:refnum<vi>)
        n166 = local read "mqtt_subscribeTopic"() -> (→"String":string)
        n167 = local read "Combo Box 2"() -> (w492:string)
        n168 = Unbundle By Name(w507) -> ("subscriptionList"=w505:string[], "ViewerRef"=w503:T9[])
        n169 = property class="Bool"(reference=w499, error in=w502, "DisabledEnum"=T17."Disabled and Grayed Out" ("Disabled")) -> (error out=w500:errorcluster)  [unwired: 1 out]
        n170 = Search 1D Array(1D array=w505, element=w492) -> (index of element=w504:i32)  [unwired: 1 in]
        n171 = case shown="-1" w504 {
          selector: w504 -> [_ w515]
          tunnel: w507 -> [w509 w524]
          tunnel: [w509 w523] -> w506
          tunnel: w505 -> [_ w522]
          tunnel: [w508 w520] -> w495
          tunnel: w503 -> [_ w518]
          tunnel: w500 -> [w508 w513]
          tunnel: w501 -> [_ w510]
          frame -1 {
          }
          frame Default {
            w519 = 1 ("length")
            # "Discard Panel VI and release\nresources"
            n172 = Delete From Array(array=w522, length=w519, index=w515) -> (deleted portion=w512:string[], array with subset deleted=w521:string[])
            n173 = Delete From Array(array=w518, length=w519, index=w515) -> (deleted portion=w516:T9[], array with subset deleted=w517:T9[])
            n174 = Bundle By Name(cluster=w524, "subscriptionList"=w521, "ViewerRef"=w517) -> (w523:T10)
            n175 = call "Send Msg and Wait on Response.vi"("error in (no error)"=w513, "Message Data"=w512, "Message"="sub_OnUnsubscribe", "Subscription References"=w510) -> ("error out"=w514:errorcluster)  [unwired: 7 in]
            n176 = disable-structure shown="Default" {
              disable-tunnel: w514 -> [w527 w531]
              disable-tunnel: [w526 w531] -> w520
              disable-tunnel: w516 -> [w525 _]
              disable-tunnel: w515 -> [_ _]
              frame condition #0 {
                n177 = for {
                  tunnel: w525 -> [w528] mode=indexing
                  shift-right: [w529] -> w526
                  shift-left: w527 -> [w530]
                  n178 = call "Delete.vi"("error in (no error)"=w530, "ViewerRef"=w528) -> ("error out"=w529:errorcluster)  [unwired: 9 in]
                }
              }
              frame condition #1 (active) {
              }
            }
          }
        }
        n179 = Unbundle By Name(w493) -> ("Subscribe"=w496:refnum<vi>)
        n180 = property class="Bool"(reference=w496, error in=w495, "DisabledEnum"=T17."Enabled" ("Disabled")) -> (error out=w494:errorcluster)  [unwired: 1 out]
      }
      frame "mqtt_unsubscribeAll" {
        # "Unsubscribe to all existing topics, if any is still active"
        n181 = Unbundle By Name(w539) -> ("ViewerRef"=w535:T9[], "subscriptionList"=w532:string[])
        n182 = Array Size(array=w532) -> (size(s)=w534:i32)
        n183 = case shown="Default" w534 {
          tunnel: w540 -> [w542 w548]
          tunnel: [w542 w550] -> w536
          tunnel: w535 -> [_ w549]
          tunnel: w532 -> [_ w543]
          tunnel: w533 -> [_ w545]
          frame 0 {
          }
          frame Default {
            n184 = call "Send Msg and Wait on Response.vi"("Priority Message? (F)"=TRUE, "error in (no error)"=w548, "Message Data"=w543, "Message"="sub_OnUnsubscribe", "Subscription References"=w545) -> ("error out"=w547:errorcluster)  [unwired: 6 in]
            n185 = disable-structure shown="PanelView==True" {
              disable-tunnel: w547 -> [w553 w557]
              disable-tunnel: [w552 w557] -> w550
              disable-tunnel: w549 -> [w551 _]
              frame condition #0 {
                n186 = for {
                  shift-right: [w555] -> w552
                  shift-left: w553 -> [w556]
                  tunnel: w551 -> [w554] mode=indexing
                  n187 = call "Delete.vi"("error in (no error)"=w556, "ViewerRef"=w554) -> ("error out"=w555:errorcluster)  [unwired: 9 in]
                }
              }
              frame condition #1 (active) {
              }
            }
          }
        }
        n188 = Bundle By Name(cluster=w539, "subscriptionList"=string[] []) -> (w538:T10)
      }
      frame "Exit" {
        # "Stop the VI"
        # "Release the message queue reference"
        # "#CodeNeeded - Add any required cleanup code here. Note that if 'Exit' was called as a result of an error, an error dialog will be displayed. Add any custom error handling for an 'Exit' condition here as well."
        # "Exit - Exit the application."
        n189 = Variant To Data(type=errorcluster {"status"=FALSE, "code"=0, "source"=""} ("error constant"), Variant=w559) -> (data=w560:errorcluster)  [unwired: 1 in, 1 out]
        n190 = call <vilib>:"Simple Error Handler.vi"("error in (no error)"=w560) -> ()  [unwired: 4 in, 5 out]
        n191 = call "Fire User Event - Stop.vi"("User Event - Stop"=w564) -> ("error out"=w563:errorcluster)  [unwired: 10 in]
        n192 = Release Queue(queue=w569, error in (no error)=w562) -> (error out=w566:errorcluster)  [unwired: 1 in, 2 out]
        n193 = Merge Errors(w563, w566) -> (w565:errorcluster)
      }
      frame Default {
        # "'Default' case only runs if there is a message that isn't defined in any of the other cases.  Output a programming error."
        n194 = xnode "Error Ring"("parameter 0"=w571) -> ("error out"=w572:errorcluster)
      }
    }
    n195 = call "Error Handler - Message Handling Loop.vi"("error in (no error)"=w274, "Ignore Errors (Runtime)"=i32[] [56], "Message Queue"=w276) -> ("dup error in"=w275:errorcluster)  [unwired: 7 in, 1 out]
  }
  n196 = while {
    tunnel: w26 -> [w590]
    shift-right: [w588] -> w23
    shift-left: w20 -> [w589]
    tunnel: [w585] -> w21
    tunnel: w3 -> [w583]
    shift-right: [w582] -> _
    shift-left: -1 -> [w581]
    stop <- w586 stop-if-true
    # "Event Handling Loop"
    n197 = event shown="[1] \"mqtt_disconnect\": Value Change" {
      selector: w589 -> [_ _ _ _ _ _ _ _ _ _ _ _]
      dyn-events: [_ _ _ _ _ _ _ _ _ _ _ _] -> w588
      timeout: w581 -> [_ _ _ _ _ _ _ _ _ _ _ _]
      tunnel: [_ _ _ _ _ _ _ _ _ _ TRUE ("Discard?") _] -> w586
      tunnel: w590 -> [w595 w600 w605 w617 w626 w631 w636 w642 w645 w649 w655 w658]
      tunnel: [w593 w598 w603 w615 w624 w629 w634 w641 _ w648 _ _] -> w587
      tunnel: [w592 w597 w602 w614 w623 w628 w633 w638 w645 w647 w655 w658] -> w584
      tunnel: w583 -> [_ _ _ _ _ _ _ _ _ _ w654 _]
      tunnel: [w591 -1 ("NewVal") w601 w613 w622 w627 w632 w637 w644 w646 w651 w657] -> w582
      tunnel: w581 -> [w591 _ w601 w613 w622 w627 w632 w637 w644 w646 w651 _]
      event "mqtt_connect": Value Change {
        # "#CodeNeeded - Send the appropriate message for this user interface event."
        n198 = event-data() -> ()  [unwired: 1 in, 1 out]
        n199 = disable-structure shown="Disabled" {
          frame Disabled {
            n200 = property on="mqtt_subscribeTopic" class="CmbBox" props=["Strings[]"]() -> ()  [unwired: 3 in, 2 out]
          }
          frame Enabled {
          }
        }
        n201 = call-poly "Enqueue Message.vi"("Message"="mqtt_connect", "Message Queue"=w595) -> ("error out"=w593:errorcluster, "dup Message Queue"=w592:refnum<queue>)  [unwired: 8 in]
      }
      event "mqtt_disconnect": Value Change {
        # "If automated messaging is turned on, turn it off"
        # "#CodeNeeded - Send the appropriate message for this user interface event."
        n202 = event-data() -> ()  [unwired: 1 in, 1 out]
        n203 = call-poly "Enqueue Message.vi"("Message"="mqtt_disconnect", "Message Queue"=w600) -> ("error out"=w598:errorcluster, "dup Message Queue"=w597:refnum<queue>)  [unwired: 8 in]
      }
      event "mqtt_publish": Value Change {
        n204 = event-data() -> ()  [unwired: 1 in, 1 out]
        n205 = call-poly "Enqueue Message.vi"("Message"="mqtt_publish", "Message Queue"=w605) -> ("error out"=w603:errorcluster, "dup Message Queue"=w602:refnum<queue>)  [unwired: 8 in]
      }
      event Timeout {
        n206 = event-data() -> ()  [unwired: 1 in, 1 out]
        n207 = Get Date/Time In Seconds() -> (seconds since 1Jan1904=w607:timestamp)
        n208 = Concatenate Strings("AM Command", " - %T" ("string")) -> (w608:string)
        n209 = Format Into String(format string=w608, w607) -> (resulting string=w606:string)  [unwired: 2 in, 1 out]
        n210 = local write "mqtt|_sendTopic"("AM Topic") -> ()
        n211 = local write "Publish Meta"("AM Publish Meta") -> ()
        n212 = local write "Command"(w606) -> ()
        n213 = flat-sequence {
          tunnel: w617 -> [w621]
          tunnel: "mqtt_publish" ("Message") -> [w620]
          tunnel: [w619] -> w615
          tunnel: [w618] -> w614
          tunnel: w606 -> [_]
          frame #0 {
            n214 = call-poly "Enqueue Message.vi"("Message"=w620, "Message Queue"=w621) -> ("error out"=w619:errorcluster, "dup Message Queue"=w618:refnum<queue>)  [unwired: 8 in]
          }
        }
      }
      event "mqtt_subscribe": Value Change {
        n215 = event-data() -> ()  [unwired: 1 in, 1 out]
        n216 = call-poly "Enqueue Message.vi"("Message"="mqtt_subscribe", "Message Queue"=w626) -> ("error out"=w624:errorcluster, "dup Message Queue"=w623:refnum<queue>)  [unwired: 8 in]
      }
      event "mqtt_unsubscribe": Value Change {
        n217 = event-data() -> ()  [unwired: 1 in, 1 out]
        n218 = call-poly "Enqueue Message.vi"("Message"="mqtt_unsubscribe", "Message Queue"=w631) -> ("error out"=w629:errorcluster, "dup Message Queue"=w628:refnum<queue>)  [unwired: 8 in]
      }
      event "Clear Console": Value Change {
        n219 = event-data() -> ()  [unwired: 1 in, 1 out]
        n220 = call-poly "Enqueue Message.vi"("Message"="ClearConsole", "Message Queue"=w636) -> ("error out"=w634:errorcluster, "dup Message Queue"=w633:refnum<queue>)  [unwired: 8 in]
      }
      event Panel Close? {
        # "Confirm quit status manages safe application shutdown"
        n221 = event-data() -> ()  [unwired: 1 in, 1 out]
        n222 = call-poly "Enqueue Message.vi"("Priority Message? (F)"=TRUE, "Message"="Confirm Quit", "Message Queue"=w642) -> ("error out"=w641:errorcluster, "dup Message Queue"=w638:refnum<queue>)  [unwired: 7 in]
        n223 = event-data("Discard?"=TRUE) -> ()  [unwired: 1 in, 1 out]
      }
      event Application Instance Close {
        # "Not implemented yet"
        # "#CodeRecommended - When a project closes, all VIs within that project are aborted and leave memory. However, any code placed in this event frame is guaranteed to run to completion, so add any cleanup code that absolutely must happen here."
        n224 = event-data() -> ()  [unwired: 1 in, 1 out]
      }
      event "Exit": Value Change {
        # "Confirm quit status manages safe application shutdown"
        n225 = event-data() -> ()  [unwired: 1 in, 1 out]
        n226 = call-poly "Enqueue Message.vi"("Message"="Confirm Quit", "Message Queue"=w649) -> ("error out"=w648:errorcluster, "dup Message Queue"=w647:refnum<queue>)  [unwired: 8 in]
      }
      event User Event {
        # "Close subscriber loop and exit"
        # "The Message Handling Loop processed an \"Exit\" message, which fired this event to stop the Event Handling Loop."
        n227 = event-data() -> ()  [unwired: 1 in, 1 out]
        n228 = Unbundle By Name(w654) -> ("SubscribeQ"=w652:refnum<queue>)
        n229 = call-poly "Enqueue Message.vi"("Message"="Exit", "Message Queue"=w652) -> ()  [unwired: 8 in, 2 out]
      }
      event "Message Period (ms)": Value Change {
        n230 = event-data() -> ("NewVal"=w657:i32)  [unwired: 1 in]
      }
    }
    n231 = call "Error Handler - Event Handling Loop.vi"("error in (no error)"=w587, "Message Queue"=w584) -> ("dup error in"=w585:errorcluster)  [unwired: 8 in, 1 out]
  }
  n232 = Unregister For Events(event registration refnum=w23, error in=w21) -> (error out=w24:errorcluster)
  n233 = Merge Errors(w24, w27, w14) -> (w25:errorcluster)
  n234 = call "Destroy User Event - Stop.vi"("error in (no error)"=w25, "User Event - Stop"=w19) -> ("error out"=w8:errorcluster)  [unwired: 9 in]
  n235 = Release Notifier(notifier=w5, error in (no error)=w8) -> (error out=w7:errorcluster)  [unwired: 1 in, 2 out]
  n236 = disable-structure shown="RUN_TIME_ENGINE==True" {
    disable-tunnel: w7 -> [_ _]
    frame condition #0 (active) {
    }
    frame condition #1 {
      # "Call Quit LabVIEW if running as a built application."
      n237 = Quit LabVIEW() -> ()  [unwired: 1 in]
    }
  }
